vi "LINC COSMOS Array Item.vi"(5 "ignore":bool, 8 "error in (no error)":errorcluster, 9 "packet fields":T1, 10 "packet index":i32, 11 "packets in":T2[](array[typedef])) -> (0 "error out":errorcluster, 2 "item index":i32, 3 "packets out":T2[](array[typedef]))   [LabVIEW 2018, in "STEPkgDriver_LINC.lvlib"]
uses:
  STEPkgDriver_LINC.lvlib
  LINC Format Prototype.ctl
  LINC Packet.ctl
  LINC Packet Fields.ctl
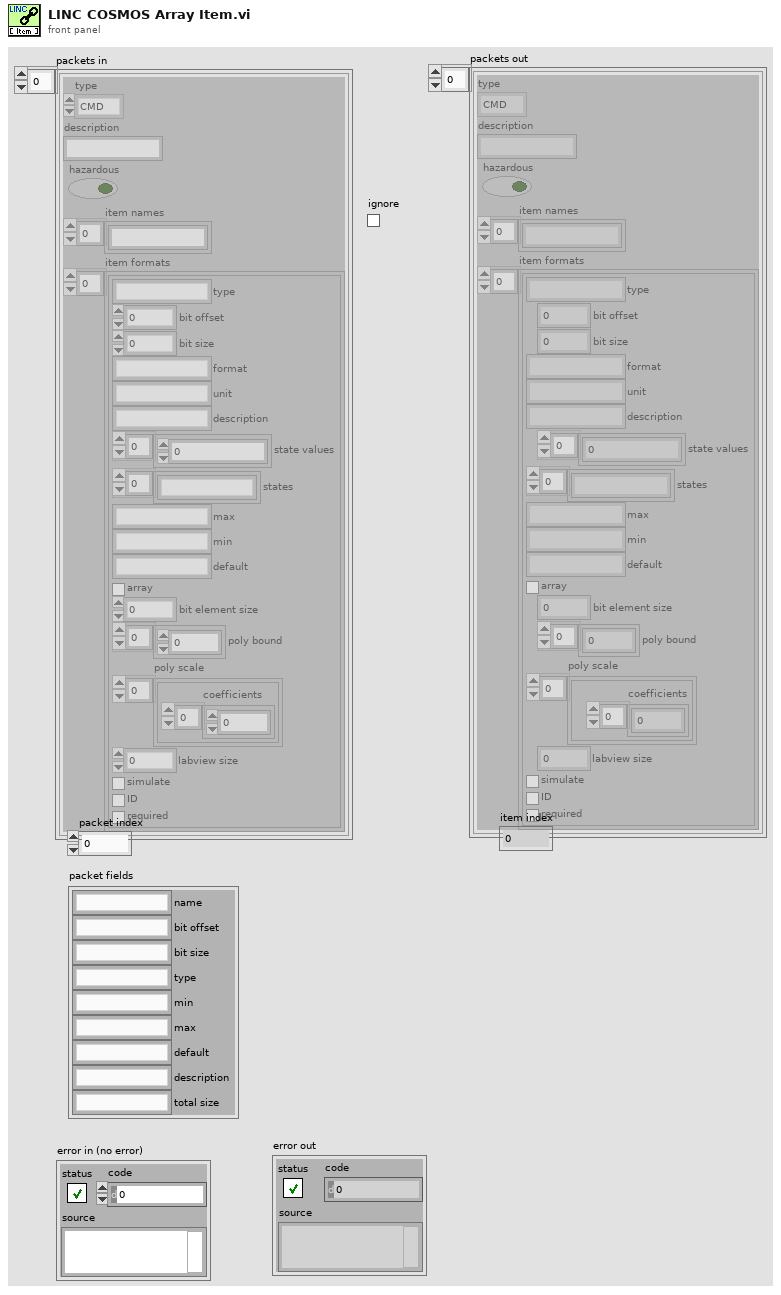
[diagram p1: front panel]
types:
  T1 = typedef "STEPkgDriver_LINC.lvlib/LINC Packet Fields.ctl" = cluster{"name":string, "bit offset":string, "bit size":string, "type":string, "min":string, "max":string, "default":string, "description":string, "total size":string}
  T2 = typedef "STEPkgDriver_LINC.lvlib/LINC Packet.ctl" = cluster{"type":enum16{"CMD", "TLM"}, "description":string, "hazardous":bool, "item names":string[], "item formats":T3[]}
  T3 = typedef "STEPkgDriver_LINC.lvlib/LINC Format Prototype.ctl" = cluster{"type":string, "bit offset":i32, "bit size":i32, "format":string, "unit":string, "description":string, "state values":i64[], "states":string[], "max":string, "min":string, "default":string, "array":bool, "bit element size":i32, "poly bound":dbl[], "poly scale":cluster{"coefficients":dbl[]}[], "labview size":i32, "simulate":bool, "ID":bool, "required":bool}
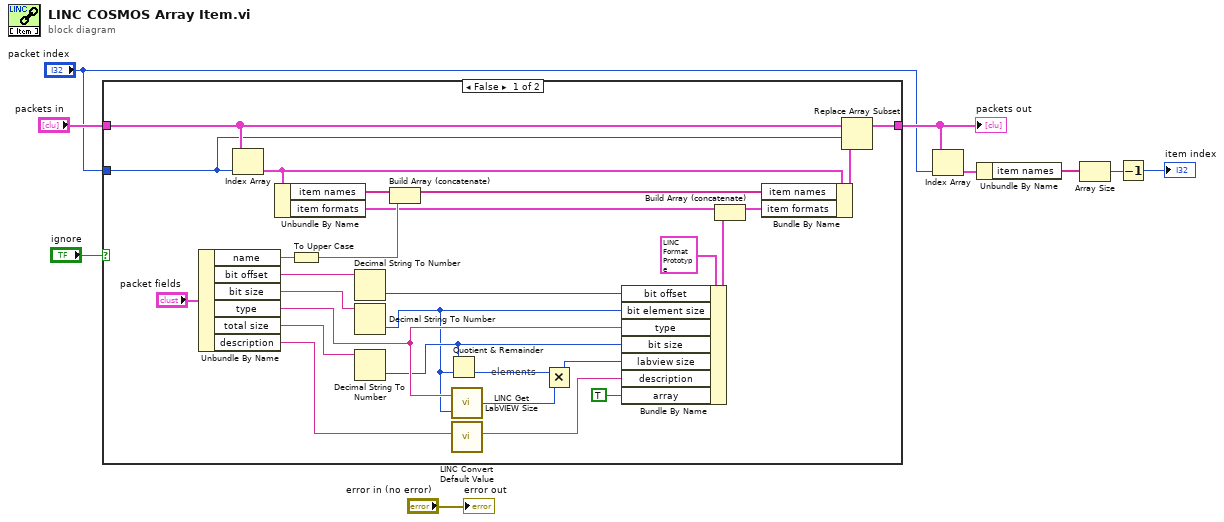
[diagram p0: block diagram]
diagram:
  n1 = case shown="False" "ignore" {
    tunnel: "packets in" -> [w25 w37]
    tunnel: [w24 w37] -> w2
    tunnel: "packet index" -> [w23 _]
    frame False {
      # "elements"
      n2 = Unbundle By Name("packet fields") -> ("name"=w21:string, "bit offset"=w20:string, "bit size"=w19:string, "type"=w18:string, "total size"=w17:string, "description"=w16:string)
      n3 = Index Array(array=w25, index=w23) -> (element=w31:T2)
      n4 = Unbundle By Name(w31) -> ("item names"=w29:string[], "item formats"=w26:T3[])
      n5 = To Upper Case(1:w21) -> (0:w33:string)
      n6 = Decimal String To Number(string=w20) -> (number=w34:i32)  [unwired: 2 in, 1 out]
      n7 = Decimal String To Number(string=w19) -> (number=w10:i32)  [unwired: 2 in, 1 out]
      n8 = Decimal String To Number(string=w17) -> (number=w14:i32)  [unwired: 2 in, 1 out]
      n9 = Build Array (concatenate)(w29, w33) -> (w28:string[])
      n10 = Quotient & Remainder(x=w14, y=w10) -> (floor(x/y)=w13:i32)  [unwired: 1 out]
      n11 = call "LINC Get LabVIEW Size.vi"("bit size"=w10, "type"=w18) -> ("labview size"=w12:i32)
      n12 = call "LINC Convert Default Value.vi"("default in"=w16) -> ("default out"=w32:string)  [unwired: 10 in]
      n13 = Multiply(x=w13, y=w12) -> (x*y=w11:i32)
      n14 = Bundle By Name(cluster=T3 {"type"="", "bit offset"=0, "bit size"=0, "format"="", "unit"="", "description"="", "state values"=[], "states"=[], "max"="", "min"="", "default"="", "array"=FALSE, "bit element size"=0, "poly bound"=[], "poly scale"=[], "labview size"=0, "simulate"=FALSE, "ID"=FALSE, "required"=FALSE} ("data"), "bit offset"=w34, "bit element size"=w10, "type"=w18, "bit size"=w14, "labview size"=w11, "description"=w32, "array"=TRUE) -> (w35:T3)
      n15 = Build Array (concatenate)(w26, w35) -> (w27:T3[])
      n16 = Bundle By Name(cluster=w31, "item names"=w28, "item formats"=w27) -> (w30:T2)
      n17 = Replace Array Subset(array=w25, new element=w30, index=w23) -> (w24:T2[])
    }
    frame True {
    }
  }
  "packets out" <- w2
  n18 = Index Array(array=w2, index="packet index") -> (element=w6:T2)
  n19 = Unbundle By Name(w6) -> ("item names"=w5:string[])
  n20 = Array Size(array=w5) -> (size(s)=w4:i32)
  n21 = Decrement(x=w4) -> (x-1=→"item index":i32)
  "error out" <- "error in (no error)"
